vi "AlazarFFTBackgroundSubtractionSetRecordS16.vi"(3 "error in (no error)":errorcluster, 4 "Record":i16[](array[numeric]), 5 "DSP Handle":u64) -> (0 "error out":errorcluster, 1 "Return Code":u32, 2 "DSP Handle":u64)   [LabVIEW 2009]
uses:
  ATSApi.dll
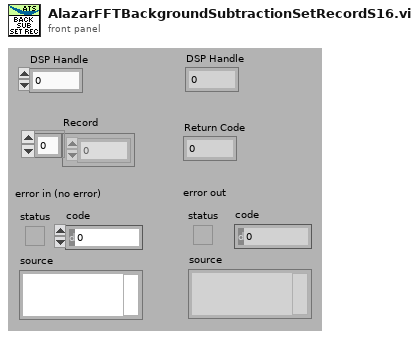
[diagram p1: front panel]
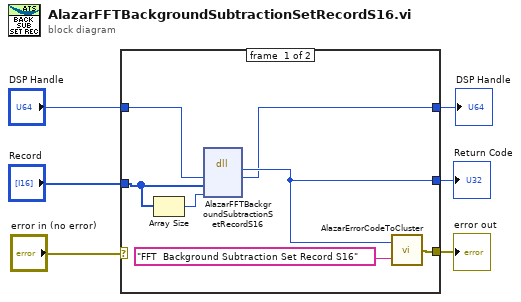
[diagram p0: block diagram]
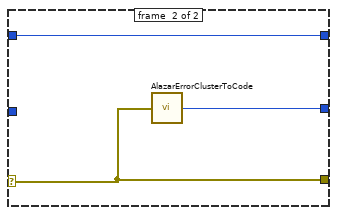
[diagram p2: hidden frame]
diagram:
  n1 = case shown="No Error" "error in (no error)" {
    selector: "error in (no error)" -> [_ w14]
    tunnel: [w10 w14] -> w5
    tunnel: [w12 w15] -> w1
    tunnel: "DSP Handle" -> [w13 w16]
    tunnel: [w9 w16] -> w3
    tunnel: "Record" -> [w8 _]
    frame #0 {
      n2 = Array Size(array=w8) -> (size(s)=w7:i32)
      n3 = dll-call lib="ATSApi.dll" fn="AlazarFFTBackgroundSubtractionSetRecordS16"("dspHandle"=w13, "record"=w8, "size_samples"=w7) -> ("return type"=w12:u32, "dspHandle"=w9:u64)  [unwired: 5 in, 2 out]
      n4 = call "AlazarErrorCodeToCluster.vi"("Message"="FFT  Background Subtraction Set Record S16", "Error Code"=w12) -> ("error out"=w10:errorcluster)
    }
    frame #1 {
      n5 = call "AlazarErrorClusterToCode.vi"("error in (no error)"=w14) -> ("Error Code"=w15:u32)
    }
  }
  "DSP Handle" <- w3
  "error out" <- w5
  "Return Code" <- w1
